vi "RT_Call Config.vi"(5 "Number of Bytes to Read":u16, 7 "Number of Bytes to Write":u16, 8 "error in":errorcluster, 10 "Command (Write & Read)":u8(ring) items=["Write & Read", "Write", "Read"], 11 "FPGA VI Reference In":T1) -> (0 "error out":errorcluster, 3 "FPGA VI Reference Out":T1)   [LabVIEW 2018]
uses:
  Data Def/RT_FPGA VI Reference.ctl
  <vilib>/Utility/error.llb/Error Cluster From Error Code.vi
  <vilib>/rvi/errors/niLvFpgaAdjustHostInterfaceError.vi
  <vilib>/rvi/interface/nirviReadWriteControl/nirviReadWriteControl.xnode
  <vilib>/rvi/interface/Simulation/niFpgaSimulationCallBeginRW.vi
  NiFpgaLv.dll
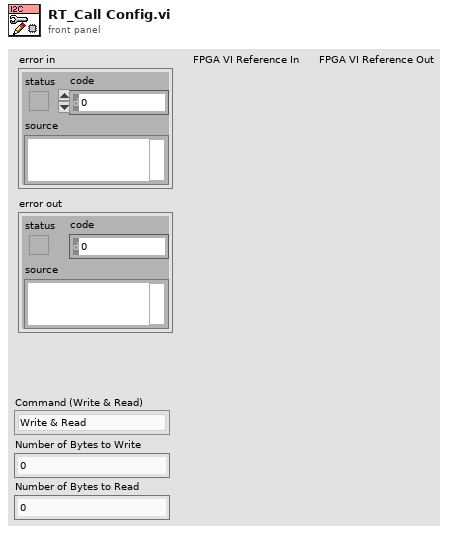
[diagram p1: front panel]
types:
  T1 = typedef "RT_FPGA VI Reference.ctl" = refnum<k20>
  T2 = enum16{"Idle", "Set Idle", "Config", "Read", "Write", "Arm", "Auto Run", "Auto Config", "Auto Write", "Auto Arm", "Auto Read", "Auto Check"}
  T3 = cluster{"Command (Write & Read)":u8, "Number of Bytes to Write":u16, "Number of Bytes to Read":u16}
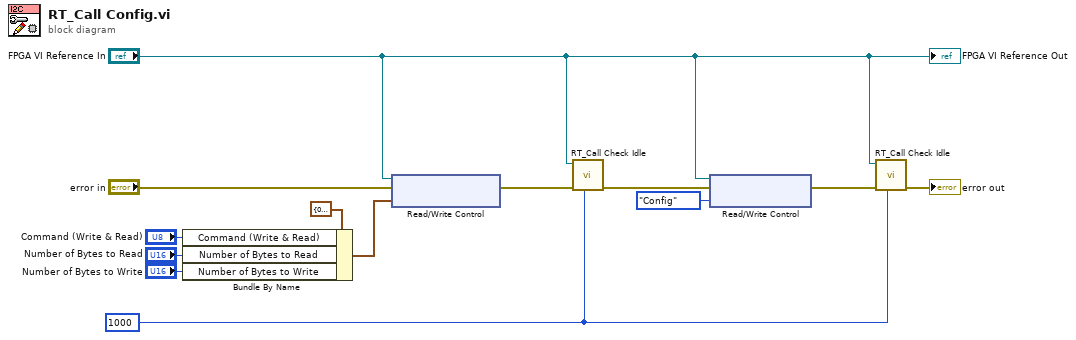
[diagram p0: block diagram]
diagram:
  w12 = 1000 ("Timeout?")
  n1 = Bundle By Name(cluster=T3 {"Command (Write & Read)"=0, "Number of Bytes to Write"=0, "Number of Bytes to Read"=0} ("Command Data"), "Command (Write & Read)"="Command (Write & Read)", "Number of Bytes to Read"="Number of Bytes to Read", "Number of Bytes to Write"="Number of Bytes to Write") -> (w2:T3)
  n2 = xnode "Read/Write Control"("FPGA VI Reference In"="FPGA VI Reference In", "error in"="error in", "Command Data"=w2) -> ("error out"=w11:errorcluster)  [unwired: 1 out]
  n3 = call "RT_Call Check Idle.vi"("Timeout?"=w12, "error in"=w11, "FPGA VI Reference In"="FPGA VI Reference In") -> ("error out"=w10:errorcluster)  [unwired: 7 in, 1 out]
  n4 = xnode "Read/Write Control"("FPGA VI Reference In"="FPGA VI Reference In", "error in"=w10, "I2C Loop State"=T2."Config") -> ("error out"=w9:errorcluster)  [unwired: 1 out]
  n5 = call "RT_Call Check Idle.vi"("Timeout?"=w12, "error in"=w9, "FPGA VI Reference In"="FPGA VI Reference In") -> ("error out"=→"error out":errorcluster)  [unwired: 7 in, 1 out]
  "FPGA VI Reference Out" <- "FPGA VI Reference In"
